vi "SVT Fractional-octave Analysis (N Ch).vi"(0 "scaled signals [EU]":waveform(dbl)[](array[waveform])=[{"t0"=timestamp(0 s since 1904-01-01), "dt"=1.0, "Y"=[]}], 1 "restart averaging (F)":bool, 2 "reset filter (F)":bool, 5 "frequency range [Hz]":T8={"low frequency"=125.0, "high frequency"=8000.0} {"high frequency" min=0.001 format="%.2f"; "low frequency" min=0.001 format="%.2f"}, 7 "bandwidth":T2(ring)=enum."1/12 octave", 9 "dB On (T)":bool=TRUE, 11 "error in (no error)":errorcluster, 12 "averaging type":T9(ring), 13 "exp avg settings":T1={" mode"=enum."Fast", "time constant [ms]"=125.0} {"time constant [ms]" format="%.2f"}, 14 "equal confidence level [dB]":dbl=125.0 format="%.2f") -> (3 "filter settled":bool, 4 "octave spectra":T7(array[cluster]) {"band power" format="%.2f"; "nominal frequencies [Hz]" format="%.2f"}, 6 "unit labels":string[](array[string]), 8 "total band powers":dbl[](array[numeric]) format="%.2f", 10 "octave info":T3[](array[typedef]) {"engineering units" items=["custom..."=0, "V"=1, "A"=21, "C"=30, "pC"=31, "s"=32, "-"=29, "Pa"=2, "N"=20, "g"=3, "m/s^2"=4, "m/s"=5, "m"=6, "mm/s"=12, "mm"=13, "micron/s"=14, "micron"=15, "in/s^2"=7, "in/s"=8, "in"=9, "mil/s"=10, "mil"=11, "rad/s^2"=16, "rad/s"=17, "rad"=18, "deg/s^2"=26, "deg/s"=27, "deg"=28, "RPM"=22, "cycle/s^2"=23, "Hz"=24, "cycle"=25, "strain"=19]; "dB reference" format="%.2e"; "weighting filter" items=["Linear", "A-weighting", "B-weighting", "C-weighting", "ITU-R 468-4", "Dolby", "CCITT", "C-message", "Wb", "Wc", "Wd", "We", "Wf", "Wh", "Wj", "Wk", "Wm", "AES17 20 kHz lowpass", "AES17 40 kHz lowpass", "AES17 20 kHz highpass", "AES17 40 kHz highpass"]}, 15 "error out":errorcluster)   [LabVIEW 2017, in "SoundVib_Octave.lvlib"]
doc: "LabVIEW no longer supports this VI. The SVT Fractional-octave Analysis VI is available for compatibility with previous versions of the LabVIEW Sound and Vibration Toolkit. This version of the SVT Fractional-octave Analysis VI performs a fractional-octave analysis on <B>scaled signal [EU]</B> in accordance with the IEC 1260 standard. This standard has been superseded by the new IEC 61260 standard. If you want to ensure compliance with the latter standard, use the SVT Fractional-octave Analysis VI, located on the Octave Analysis palette instead. You can use this polymorphic VI to perform fractional-octave analysis on a single channel or on N channels. The data type you wire to the <B>scaled signal [EU]</B> input determines the polymorphic instance to use."
uses:
  <vilib>/addons/Sound and Vibration/svt_Octave/SoundVib_Octave.lvlib
  <vilib>/addons/_NISVFA/_Shared subVIs/Controls/svc_Octave Info.ctl
  <vilib>/addons/_NISVFA/_Shared subVIs/Controls/svc_Octave Standard.ctl
  <vilib>/addons/_NISVFA/_Shared subVIs/Controls/svc_Weighting Filter Text Ring.ctl
  <vilib>/addons/_NISVFA/_Shared subVIs/Controls/svc_Engineering Units Text Ring.ctl
  <vilib>/addons/Sound and Vibration/svt_Octave_2014 standard/SoundVib_Octave_2014 standard.lvlib
panel:
  out "# samples to settle":u64
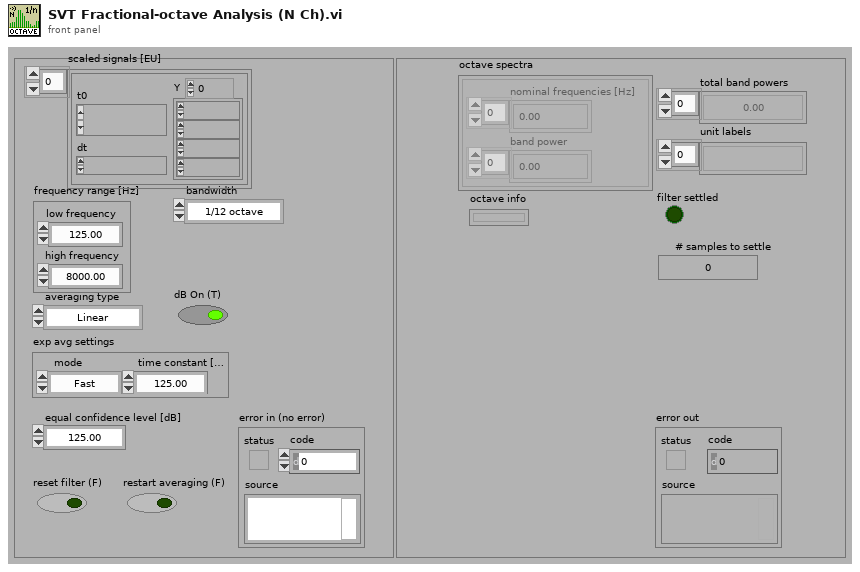
[diagram p1: front panel]
types:
  T1 = cluster{" mode":enum16{"Slow", "Fast", "Impulse", "Custom"}, "time constant [ms]":dbl}
  T2 = enum16{"1 octave", "1/3 octave", "1/6 octave", "1/12 octave", "1/24 octave"}
  T3 = typedef "svc_Octave Info.ctl" = cluster{"standard":T4, "bandwidth":enum16{"1 octave", "1/3 octave", "1/6 octave", "1/12 octave", "1/24 octave"}, "low band":i32, "high band":i32, "weighting filter":T5, "dB reference":dbl, "dB On":bool, "unit label":string, "channel name":string, "description":string, "engineering units":T6, "custom label":string, "spectrum type":enum16{"power", "magnitude"}, "spectral density":bool, "filters settled":bool}
  T4 = typedef "svc_Octave Standard.ctl" = enum16{"ANSI S1.11", "IEC 61260"}
  T5 = typedef "svc_Weighting Filter Text Ring.ctl" = u16
  T6 = typedef "svc_Engineering Units Text Ring.ctl" = u16
  T7 = cluster{"nominal frequencies [Hz]":dbl[], "band power":dbl[]}[]
  T8 = cluster{"low frequency":dbl, "high frequency":dbl}
  T9 = enum16{"Linear", "Exponential", "Equal confidence", "Peak"}
  T10 = cluster{"standard":T4, "bandwidth":enum16{"1 octave", "1/3 octave", "1/6 octave", "1/12 octave", "1/24 octave"}}
  T11 = cluster{"dup nominal frequencies [Hz":dbl[], "band power [EU^2 rms]":dbl[]}[]
  T12 = cluster{"nominal frequencies [Hz]":dbl[], "band power [dB EU]":dbl[]}[]
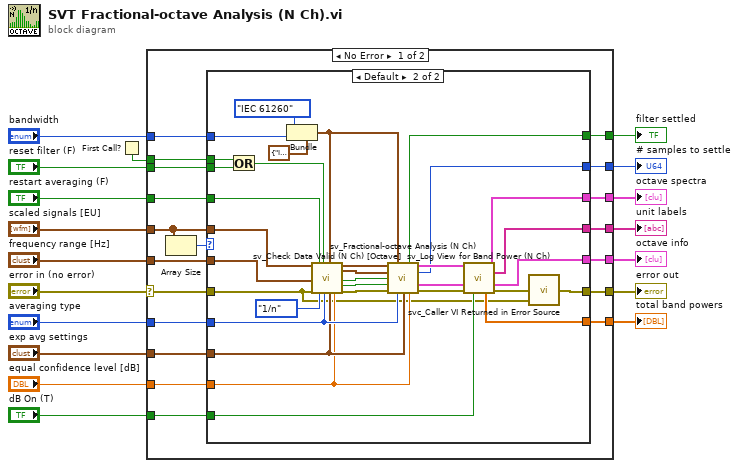
[diagram p0: block diagram]
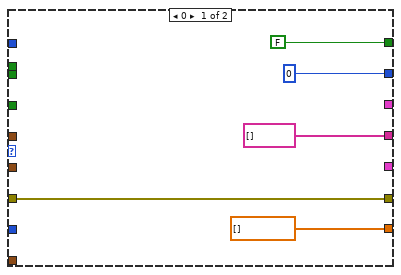
[diagram p2: hidden frame]
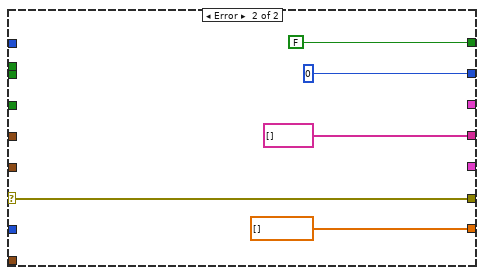
[diagram p3: hidden frame]
diagram:
  n1 = First Call?() -> (First Call?: T/F=w2:bool)
  n2 = case shown="No Error" "error in (no error)" {
    selector: "error in (no error)" -> [w27 w79]
    tunnel: "restart averaging (F)" -> [w37 _]
    tunnel: [w25 FALSE ("settled?")] -> w17
    tunnel: "dB On (T)" -> [w36 _]
    tunnel: "averaging type" -> [w35 _]
    tunnel: [w34 dbl[] [] ("total band power(s) [dB EU]")] -> w14
    tunnel: "equal confidence level [dB]" -> [w26 _]
    tunnel: "bandwidth" -> [w33 _]
    tunnel: "frequency range [Hz]" -> [w32 _]
    tunnel: "exp avg settings" -> [w31 _]
    tunnel: "scaled signals [EU]" -> [w20 _]
    tunnel: [w22 w79] -> w8
    tunnel: [w30 _] -> w7
    tunnel: [w29 _] -> w6
    tunnel: [w28 string[] [] ("unit labels")] -> w5
    tunnel: "reset filter (F)" -> [w24 _]
    tunnel: w2 -> [w23 _]
    tunnel: [w21 u64 0 ("# samples to settle")] -> w1
    frame No Error {
      n3 = Array Size(array=w20) -> (size(s)=w19:i32)
      n4 = case shown="Default" w19 {
        tunnel: w37 -> [_ w74]
        tunnel: w36 -> [_ w69]
        tunnel: w35 -> [_ w67]
        tunnel: [dbl[] [] ("total band power(s) [dB EU]") w66] -> w34
        tunnel: w33 -> [_ w44]
        tunnel: w32 -> [_ w64]
        tunnel: w31 -> [_ w63]
        tunnel: w20 -> [_ w62]
        tunnel: [_ w61] -> w30
        tunnel: [_ w60] -> w29
        tunnel: [string[] [] ("unit labels") w59] -> w28
        tunnel: w27 -> [w41 w47]
        tunnel: w26 -> [_ w55]
        tunnel: [FALSE ("settled?") w53] -> w25
        tunnel: w24 -> [_ w52]
        tunnel: w23 -> [_ w51]
        tunnel: [w41 w49] -> w22
        tunnel: [u64 0 ("# samples to settle") w48] -> w21
        frame 0 {
        }
        frame Default {
          n5 = Or(x=w51, y=w52) -> (x .or. y?=w56:bool)
          n6 = Bundle(cluster=T10 {"standard"=enum."IEC 61260", "bandwidth"=enum."1/3 octave"} ("1/n Octave settings"), "standard"=svc_Octave_Standard."IEC 61260", "bandwidth"=w44) -> (w43:T10)
          n7 = call <vilib>:"sv_Check Data Valid (N Ch) [Octave].vi"("Scaled signal(s)"=w62, "frequency range [Hz]"=w64, "error in (no error)"=w47, "restart averaging (F)"=w74, "bandwidth"=enum16{"1/1", "1/3", "1/n"}."1/n", "reset filter (F)"=w56, "averaging type"=w67, "1/n Octave settings"=w43, "exp avg settings"=w63, "equal confidence level [dB]"=w55) -> ("dup Scaled signal(s)"=w70:waveform(dbl)[], "band number"=w65:cluster{"low band":i32, "high band":i32}, "Restart averaging"=w72:bool, "Reset Filter"=w54:bool, "error out"=w73:errorcluster)  [unwired: 5 in]
          n8 = call <vilib>:"sv_Fractional-octave Analysis (N Ch).vi"("Scaled signal(s)"=w70, "1/n octave settings"=w43, "band number"=w65, "restart averaging (F)"=w72, "reset filter (F)"=w54, "error in (no error)"=w73, "averaging type"=w67, "exp avg settings"=w63, "equal confidence level [dB]"=w55) -> ("settled?"=w53:bool, "Octave measurements"=w68:T11, "# samples to settle"=w48:u64, "octave info"=w58:T3[], "error out"=w71:errorcluster)  [unwired: 2 in]
          n9 = call <vilib>:"sv_Log View for Band Power (N Ch).vi"("Octave measurements"=w68, "octave info"=w58, "error in (no error)"=w71, "dB On (T)"=w69) -> ("octave spectra"=w60:T12, "unit labels"=w59:string[], "octave info"=w61:T3[], "total band power(s) [dB EU]"=w66:dbl[], "error out"=w50:errorcluster)  [unwired: 7 in]
          n10 = call <vilib>:"svc_Caller VI Returned in Error Source.vi"("warning input to caller"=w47, "error in (no error)"=w50) -> ("error out"=w49:errorcluster)  [unwired: 3 in]
        }
      }
    }
    frame Error {
    }
  }
  "filter settled" <- w17
  "unit labels" <- w5
  "total band powers" <- w14
  "error out" <- w8
  "octave spectra" <- w6
  "octave info" <- w7
  "# samples to settle" <- w1
